vi "Create TCP Stream Initiator.vi"(9 "Local Port (0)":u16, 10 "Remote Port":u16, 11 "Remote Address":string) -> (3 "TCP Stream Initiator":refnum<class "TCP Stream Initiator.lvclass">)   [LabVIEW 2020, in "TCP Stream Initiator.lvclass"]
doc: "Use this method to configure a TCP Stream initiator with the IP address and port of its remote counterpart."
uses:
  TCP Stream Initiator.lvclass
  G:/Utilisateurs/hugofroylan.aragon/Documents/PyCharm/neuro/labview/Nested Endpoint Actors/Protocols/TCP Strategy/TCP Stream/TCP Stream.lvclass
  TCP Stream/TCP Stream.lvclass/TCP Stream.ctl
  TCP Stream/TCP Stream.lvclass
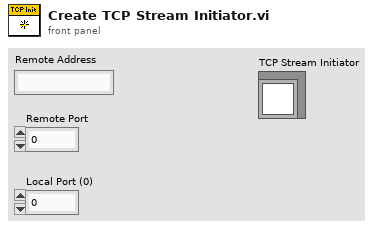
[diagram p1: front panel]
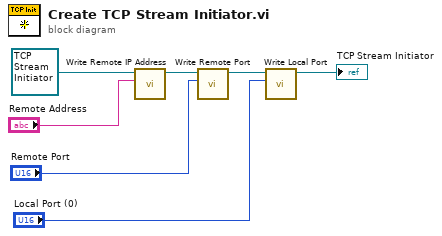
[diagram p0: block diagram]
diagram:
  n1 = call "Write Remote IP Address.vi"("Remote IP"="Remote Address", "TCP Stream in"=refnum<class "TCP Stream Initiator.lvclass"> refnum ("TCP Stream Initiator")) -> ("TCP Stream out"=w6:refnum<class "TCP Stream Initiator.lvclass">)  [unwired: 9 in]
  n2 = call "Write Remote Port.vi"("remote port"="Remote Port", "TCP Stream in"=w6) -> ("TCP Stream out"=w3:refnum<class "TCP Stream Initiator.lvclass">)  [unwired: 9 in]
  n3 = call "Write Local Port.vi"("local port"="Local Port (0)", "TCP Stream in"=w3) -> ("TCP Stream out"=→"TCP Stream Initiator":refnum<class "TCP Stream Initiator.lvclass">)  [unwired: 9 in]
